vi "Test Active Object.vi"() -> ()   [LabVIEW 2011]
uses:
  Interprocess Messenger/Send/Send.lvclass
  Interprocess Messenger/TextVarientMessage/MSG.lvclass
  Interprocess Messenger/TextVarientMessage/Extract Text (static).vi
  Interprocess Messenger/QueueMessenger/QueueMessenger.lvclass
  Interprocess Messenger/Send/Send (no data).vi
  Interprocess Messenger/Send/Send Variant.vi
  Parallel Process/PP Template (Receive type)/PP Template.lvclass
  Parallel Process/Messsage Logger/Message Logger.lvclass
  Messenging.lvlib
  Parallel Process/Attach Observer.vi
  Parallel Process/Parallel Process.lvclass
  Interprocess Messenger/Messenger (Parent)/Attach Observer.vi
  Interprocess Messenger/Messenger (Parent)/MGR.lvclass
  Parallel Process/ObserverRegister/ObserverRegistry.lvclass
  Interprocess Messenger/Send/Query (no data sent).vi
  Interprocess Messenger/SendOnly/Observer.lvclass
panel:
  out "Time (ObsSync)":string
  in  "stop":bool
  out "Time(Async)":string
  out "Time (Sync)":string
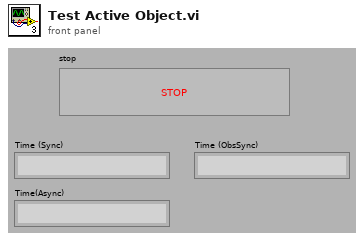
[diagram p1: front panel]
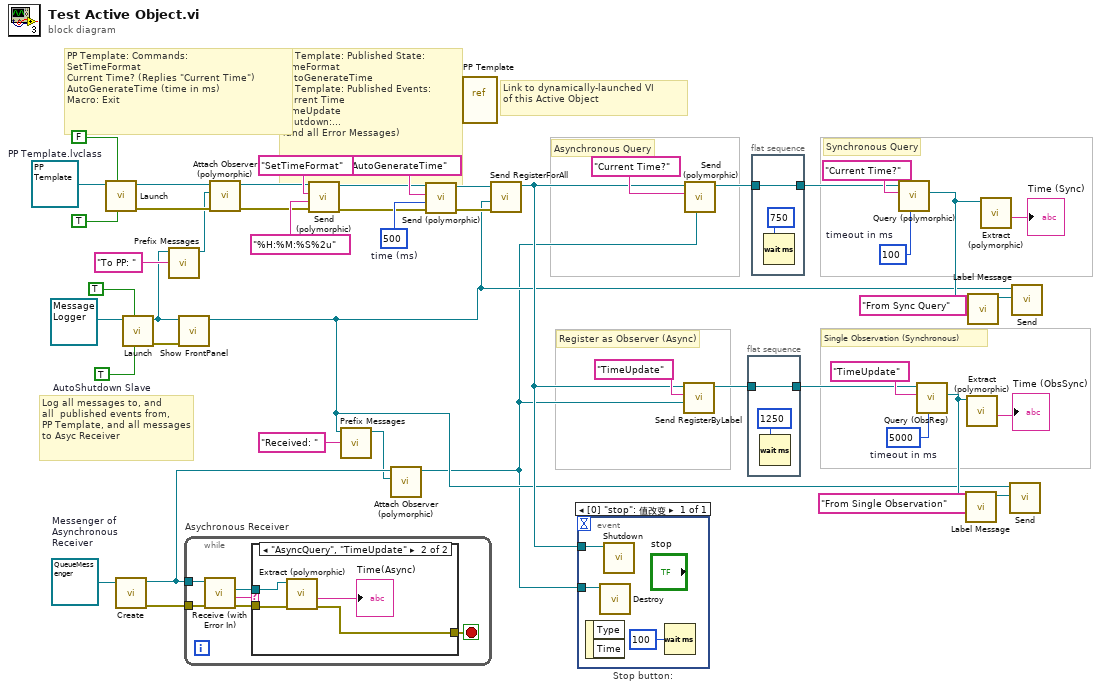
[diagram p0: block diagram]
diagram:
  w21 = 5000  # timeout in ms
  w37 = TRUE  # AutoShutdown Slave
  w41 = 500  # time (ms)
  w43 = refnum<class "QueueMessenger.lvclass"> refnum  # Messenger of Asynchronous Receiver
  w46 = 100  # timeout in ms
  w47 = refnum<class "PP Template.lvclass"> refnum  # PP Template.lvclass
  # "Single Observation (Synchronous)"
  # "PP Template: Published State:\nTimeFormat\nAutoGenerateTime\nPP Template: Published Events:\nCurrent Time\nTimeUpdate\nShutdown:...\n(and all Error Messages)"
  # "PP Template: Commands:\nSetTimeFormat\nCurrent Time? (Replies \"Current Time\")\nAutoGenerateTime (time in ms)\nMacro: Exit"
  # "Link to dynamically-launched VI\nof this Active Object"
  # "Log all messages to, and\nall  published events from,\nPP Template, and all messages\nto Asyc Receiver"
  # "Register as Observer (Async)"
  # "Asynchronous Query"
  # "Synchronous Query"
  n1 = call-dynamic "Launch.vi"("AutoShutdown Slave (F)"=TRUE, "Clone if Reentrant (T)"=FALSE, "Parallel Process in"=w47) -> ("error out"=w32:errorcluster, "Parallel Process out"=w17:refnum<class "PP Template.lvclass">)  [unwired: 1 in, 6 out]
  n2 = call-dynamic "Create.vi"("QueueMessenger in"=w43) -> ("error out"=w38:errorcluster, "QueueMessenger out"=w34:refnum<class "QueueMessenger.lvclass">)  [unwired: 1 in, 8 out]
  n3 = call-dynamic "Launch.vi"("AutoShutdown Slave (F)"=w37, "Clone if Reentrant (T)"=TRUE, "Parallel Process in"=refnum<class "Message Logger.lvclass"> refnum ("Parallel Process.lvlib:Messsage Logger.lvclass")) -> ("error out"=w40:errorcluster, "Parallel Process out"=w18:refnum<class "Message Logger.lvclass">)  [unwired: 1 in, 6 out]
  n4 = call "Prefix Messages.vi"("Prefix message labels with"="To PP: " ("Prefix to Add to Label"), "Send IN"=w18) -> ("Observer"=w15:refnum<class "Observer.lvclass">)  [unwired: 2 in, 7 out]
  n5 = call-dynamic "Show FrontPanel.vi"("error in (no error)"=w40, "Parallel Process in"=w18) -> ("Parallel Process out"=w7:refnum<class "Message Logger.lvclass">)  [unwired: 1 in, 8 out]
  n6 = while "Asychronous Receiver" {
    tunnel: w34 -> [w53]
    tunnel: w38 -> [w48]
    stop <- w49 stop-if-true
    n7 = call-dynamic "Receive (with Error In).vi"("error in (no error)"=w48, "MGR in"=w53) -> ("error out"=w52:errorcluster, "Label"=w50:string, "Message"=w51:refnum<class "MSG.lvclass">)  [unwired: 1 in, 6 out]
    n8 = case shown="\"AsyncQuery\", \"TimeUpdate\"" w50 {
      tunnel: w52 -> [w54 w58]
      tunnel: w51 -> [_ w57]
      tunnel: [w54 w56] -> w49
      frame "False", Default {
      }
      frame "AsyncQuery", "TimeUpdate" {
        n9 = call-poly "Extract (polymorphic).vi"("error in (no error)"=w58, "TextMessage in"=w57) -> ("error out"=w56:errorcluster, "Text"=→"Time(Async)":string)  [unwired: 8 out]
      }
    }
  }
  n10 = call-poly "Attach Observer (polymorphic).vi"("Observer(s)"=w15, "Parallel Process in"=w17) -> ("Parallel Process out"=w16:refnum<class "PP Template.lvclass">)  [unwired: 1 in, 8 out]
  n11 = call-poly "Send (polymorphic).vi"("error in (no error)"=w32, "Varient"="%H:%M:%S%2u" ("Label"), "Label"="SetTimeFormat", "MSR Parent in"=w16) -> ("error out"=w24:errorcluster, "MSR Parent out"=w25:refnum<class "PP Template.lvclass">)  [unwired: 6 out]
  n12 = call "Prefix Messages.vi"("Prefix message labels with"="Received: " ("Prefix to Add to Label"), "Send IN"=w7) -> ("Observer"=w33:refnum<class "Observer.lvclass">)  [unwired: 1 in, 8 out]
  n13 = call-poly "Attach Observer (polymorphic).vi"("Observer(s)"=w33, "MGR.lvclass in"=w34) -> ("MGR.lvclass out"=w6:refnum<class "QueueMessenger.lvclass">)  [unwired: 1 in, 8 out]
  n14 = call-poly "Send (polymorphic).vi"("error in (no error)"=w24, "Varient"=w41, "Label"="AutoGenerateTime", "MSR Parent in"=w25) -> ("error out"=w19:errorcluster, "MSR Parent out"=w20:refnum<class "PP Template.lvclass">)  [unwired: 6 out]
  n15 = vi-ref "PP Template.vi"() -> ()  [unwired: 1 out]
  n16 = call "Send RegisterForAll.vi"("error in (no error)"=w19, "Observer to Register"=w7, "MSR Parent in"=w20) -> ("MSR Parent out"=w8:refnum<class "PP Template.lvclass">)  [unwired: 1 in, 7 out]
  n17 = event "Stop button:" shown="[0] \"stop\": 值改变" {
    selector: _ -> [_]
    dyn-events: _ -> [_]
    timeout: _ -> [_]
    tunnel: w6 -> [w61]
    tunnel: w8 -> [w60]
    event "stop": Value Change {
      n18 = event-data() -> ()  [unwired: 3 out]
      n19 = call-dynamic "Destroy.vi"("QueueMessenger in"=w61) -> ()  [unwired: 1 in, 10 out]
      n20 = call-dynamic "Shutdown.vi"("Parallel Process in"=w60) -> ()  [unwired: 3 in, 8 out]
      n21 = Wait (ms)(milliseconds to wait=u32 100) -> ()  [unwired: 1 out]
    }
  }
  n22 = call "Send RegisterByLabel.vi"("Observer to Register"=w6, "Label"="TimeUpdate", "MSR Parent in"=w8) -> ("MSR Parent out"=w3:refnum<class "PP Template.lvclass">)  [unwired: 1 in, 7 out]
  n23 = call-poly "Send (polymorphic).vi"("Reply to..."=w6, "Label"="Current Time?", "MSR Parent in"=w8) -> ("MSR Parent out"=w5:refnum<class "PP Template.lvclass">)  [unwired: 1 in, 7 out]
  n24 = flat-sequence {
    tunnel: w3 -> [w62]
    tunnel: [w62] -> w2
    frame #0 {
      n25 = Wait (ms)(milliseconds to wait=u32 1250) -> ()  [unwired: 1 out]
    }
  }
  n26 = flat-sequence {
    tunnel: w5 -> [w64]
    tunnel: [w64] -> w4
    frame #0 {
      n27 = Wait (ms)(milliseconds to wait=u32 750) -> ()  [unwired: 1 out]
    }
  }
  n28 = call-poly "Query (polymorphic).vi"("timeout in ms (5000)"=w46, "Label"="Current Time?", "MSR Parent"=w4) -> ("Reply"=w14:refnum<class "MSG.lvclass">)  [unwired: 2 in, 6 out]
  n29 = call "Query (ObsReg).vi"("timeout in ms (5000)"=w21, "Label"="TimeUpdate", "Send"=w2) -> ("Reply"=w10:refnum<class "MSG.lvclass">)  [unwired: 1 in, 7 out]
  n30 = call-dynamic "Label Message.vi"("Label"="From Single Observation", "Message"=w10) -> ("Message"=w11:refnum<class "MSG.lvclass">)  [unwired: 1 in, 8 out]
  n31 = call-poly "Extract (polymorphic).vi"("TextMessage in"=w10) -> ("Text"=→"Time (ObsSync)":string)  [unwired: 1 in, 9 out]
  n32 = call-dynamic "Label Message.vi"("Label"="From Sync Query", "Message"=w14) -> ("Message"=w13:refnum<class "MSG.lvclass">)  [unwired: 1 in, 8 out]
  n33 = call-poly "Extract (polymorphic).vi"("TextMessage in"=w14) -> ("Text"=→"Time (Sync)":string)  [unwired: 1 in, 9 out]
  n34 = call-dynamic "Send.vi"("Message"=w11, "Message Logger in"=w7) -> ()  [unwired: 1 in, 9 out]
  n35 = call-dynamic "Send.vi"("Message"=w13, "Message Logger in"=w7) -> ()  [unwired: 1 in, 9 out]
